vi "main.vi"() -> ()   [LabVIEW 2013]
uses:
  <vilib>/picture/3D Picture Control/NI_3D Picture Control.lvlib
panel:
  out "Angle":sgl caption="角"
  out "Axis":cluster{"X":sgl, "Y":sgl, "Z":sgl} caption="轴"
  in  "Angle 9":i32(slide) scale=-730.0..730.0
  in  "Angle 7":i32(slide) scale=-50.0..200.0
  in  "Angle 8":i32(slide) scale=0.0..360.0
  in  "停止按钮":bool
  in  "Angle 6":i32(slide) scale=0.0..360.0
  out "Display":refnum<vi>(3d-picture)
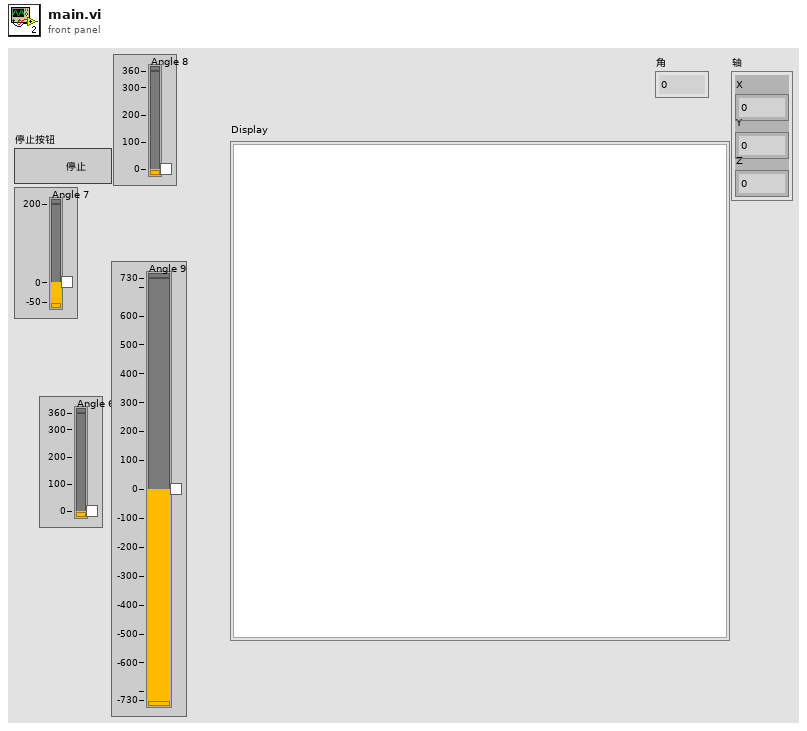
[diagram p1: front panel]
types:
  T1 = cluster{"zuoqian1":refnum<vi>, "zuoqian2":refnum<vi>, "zuoqian3":refnum<vi>}
  T2 = cluster{"zuohou1":refnum<vi>, "zuohou2":refnum<vi>, "zuohou3":refnum<vi>}
  T3 = cluster{"youqian1":refnum<vi>, "youqian2":refnum<vi>, "youqian3":refnum<vi>}
  T4 = cluster{"youhou1":refnum<vi>, "youhou2":refnum<vi>, "youhou3":refnum<vi>}
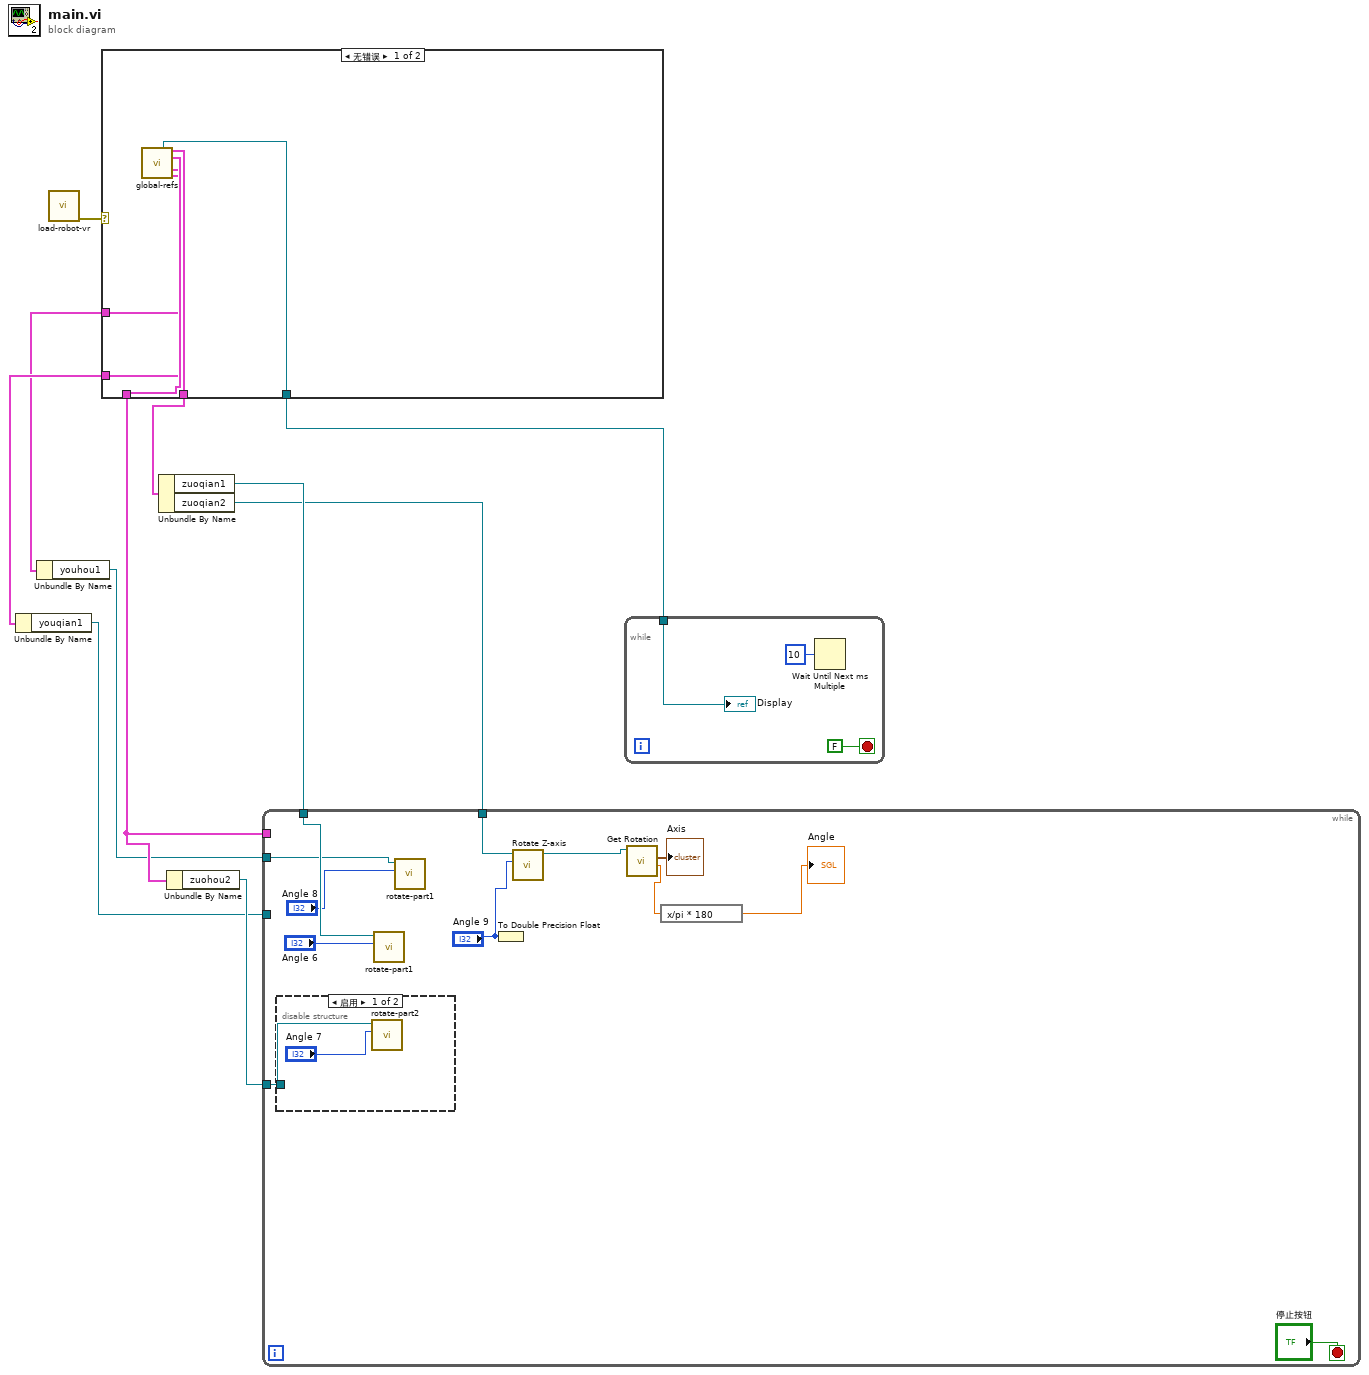
[diagram p0: block diagram]
diagram:
  n1 = call "load-robot-vr.vi"() -> ("错误输出"=w11:errorcluster)  [unwired: 11 in]
  n2 = case shown="无错误" w11 {
    tunnel: [w16 _] -> w2
    tunnel: [w15 _] -> w10
    tunnel: [w14 _] -> w9
    tunnel: [w13 _] -> w6
    tunnel: [w12 _] -> w4
    frame No Error {
      n3 = call "global-refs.vi"() -> ("RobotRef"=w16:refnum<vi>, "ZuoQianRef"=w15:T1, "ZuoHouRef"=w14:T2, "YouQianRef"=w13:T3, "YouHouRef"=w12:T4)  [unwired: 10 in, 1 out]
    }
    frame Error {
    }
  }
  n4 = Unbundle By Name(w6) -> ("youqian1"=w5:refnum<vi>)
  n5 = Unbundle By Name(w4) -> ("youhou1"=w3:refnum<vi>)
  n6 = Unbundle By Name(w10) -> ("zuoqian1"=w7:refnum<vi>, "zuoqian2"=w1:refnum<vi>)
  n7 = Unbundle By Name(w9) -> ("zuohou2"=w8:refnum<vi>)
  n8 = while {
    tunnel: w9 -> [_]
    tunnel: w8 -> [w23]
    tunnel: w7 -> [w26]
    tunnel: w5 -> [_]
    tunnel: w3 -> [w24]
    tunnel: w1 -> [w22]
    stop <- "停止按钮" stop-if-true
    n9 = disable-structure shown="启用" {
      disable-tunnel: w23 -> [w30 _]
      frame Enabled {
        n10 = call "rotate-part2.vi"("Angle"="Angle 7", "SceneObject输入"=w30) -> ()  [unwired: 10 in]
      }
      frame Disabled {
      }
    }
    n11 = call "rotate-part1.vi"("Angle"="Angle 6", "SceneObject输入"=w26) -> ()  [unwired: 10 in]
    n12 = call "rotate-part1.vi"("Angle"="Angle 8", "SceneObject输入"=w24) -> ()  [unwired: 10 in]
    n13 = To Double Precision Float(number="Angle 9") -> ()  [unwired: 1 out]
    n14 = call <vilib>:"Rotate Z-axis.vi"("angle"="Angle 9", "Scene Object In"=w22) -> ("Scene Object Out"=w20:refnum<vi>)  [unwired: 8 in, 1 out]
    n15 = call <vilib>:"Get Rotation.vi"("Scene Object"=w20) -> ("Angle"=w18:sgl, "Axis"=→"Axis":cluster{"X":sgl, "Y":sgl, "Z":sgl})  [unwired: 7 in, 2 out]
    n16 = expression code="x/pi * 180"(w18) -> (→"Angle":sgl)
  }
  n17 = while {
    tunnel: w2 -> [w33]
    stop <- FALSE stop-if-true
    n18 = Wait Until Next ms Multiple(millisecond multiple=u32 10 ("毫秒倍数")) -> ()  [unwired: 1 out]
    "Display" <- w33
  }
